vi "Keith 7001 Scan Example.vi"() -> ()   [LabVIEW 2019]
doc: "This is an example VI for the Keithley 7001 Switch System. The VI allows the operator to specify which cards are present and what channels are to be scanned. All the sources are set to immediate. The delay period applies to the trigger layer and occurs after each channel in the list is closed. After all the channels in the list have been closed, the 7001 will return to idle.\n By default this example scans channels 1 to 10 on card 1 with a 1 second delay after each channel closure."
uses:
  Keith 7001 Open/Close Chan.vi
panel:
  in  "delay period (sec)":dbl=1.0 min=0.0 max=99999.999 format="%.3f"
  out "error out":T1
  in  "error in":T1
  in  "channel list":T2(array[cluster])=[{"slot/memory"=1, "channel/row"=1, "column"=1, FALSE, FALSE}, {"slot/memory"=1, "channel/row"=2, "column"=1, FALSE, FALSE}, {"slot/memory"=1, "channel/row"=3, "column"=1, FALSE, FALSE}, {"slot/memory"=1, "channel/row"=4, "column"=1, FALSE, FALSE}, {"slot/memory"=1, "channel/row"=5, "column"=1, FALSE, FALSE}, {"slot/memory"=1, "channel/row"=6, "column"=1, FALSE, FALSE}, {"slot/memory"=1, "channel/row"=7, "column"=1, FALSE, FALSE}, {"slot/memory"=1, "channel/row"=8, "column"=1, FALSE, FALSE}, {"slot/memory"=1, "channel/row"=9, "column"=1, FALSE, FALSE}, {"slot/memory"=1, "channel/row"=10, "column"=1, FALSE, FALSE}] {"column" min=1; "channel/row" min=1; "slot/memory" min=1 max=2}
  in  "slot 2 card type (default:0)":u16(ring) items=["default", "none", "7052", "7053", "7054", "7056", "7057", "7058", "7062", "7063", "7064", "7065", "7066", "7067", "7154", "7156", "7158", "7164", "7166", "7168", "9990", "9991"]
  in  "slot 1 card type (default:0)":u16(ring) items=["default", "none", "7052", "7053", "7054", "7056", "7057", "7058", "7062", "7063", "7064", "7065", "7066", "7067", "7154", "7156", "7158", "7164", "7166", "7168", "9990", "9991"]
  in  "GPIB address":string="7"
  # "© Copyright 1993 National Instruments Corporation.  All Rights Reserved."
  # "memory location\nstandard channel"
  # "matrix card\nnon-matrix card"
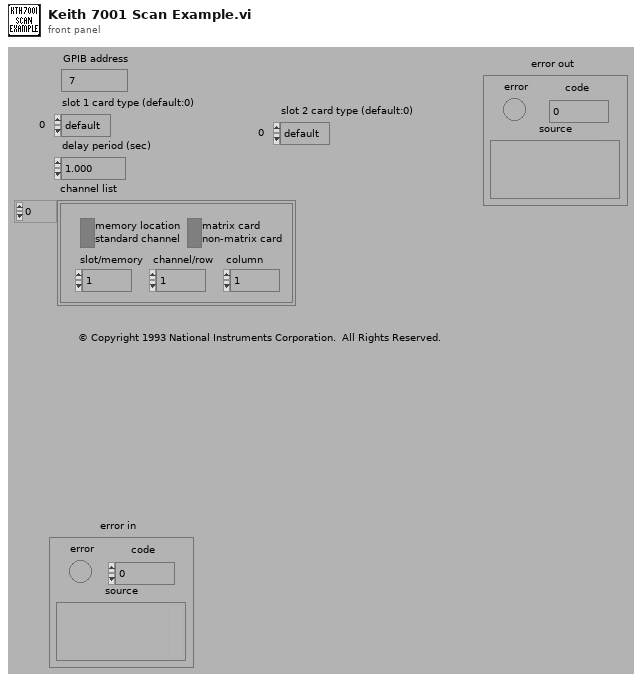
[diagram p1: front panel]
types:
  T1 = cluster{"error":bool, "code":i32, "source":string}
  T2 = cluster{"slot/memory":i16, "channel/row":i16, "column":i16, bool, bool}[]
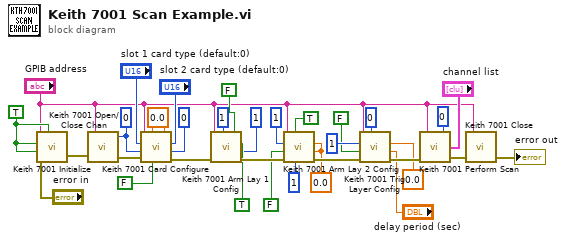
[diagram p0: block diagram]
diagram:
  w13 = 0.0
  w30 = 0.0
  w20 = u16 0
  w10 = TRUE
  n1 = call "Keith 7001 Initialize.vi"("GPIB address in"="GPIB address", "ID query"=w10, "reset"=w10, "error in"="error in", "error query"=w10) -> ("error out"=w22:T1)  [unwired: 1 out]
  n2 = call "Keith 7001 Open/Close Chan.vi"("GPIB address"="GPIB address", "error in"=w22, "open/close (open all:0)"=w20) -> ("error out"=w21:T1)  [unwired: 1 in]
  n3 = call "Keith 7001 Card Configure.vi"("slot 2 # of poles (default:0)"=u16 0, "slot 2 card type (default:0)"="slot 2 card type (default:0)", "slot 2 delay (sec)"=w30, "card pairing"=FALSE, "slot 1 delay (sec)"=w30, "error in"=w21, "slot 1 # of poles (default:0)"=w20, "slot 1 card type (default:0)"="slot 1 card type (default:0)", "GPIB address"="GPIB address") -> ("error out"=w31:T1)
  n4 = call "Keith 7001 Arm Lay 1 Config.vi"("count value"=u16 1, "count"=TRUE, "source bypass"=FALSE, "source (immediate:1)"=u16 1, "error in"=w31, "GPIB address"="GPIB address") -> ("error out"=w33:T1)  [unwired: 2 in]
  n5 = call "Keith 7001 Arm Lay 2 Config.vi"("delay period (sec)"=w13, "timer interval (sec)"=w13, "count value"=u16 1, "count"=TRUE, "error in"=w33, "source bypass"=FALSE, "source (immediate:1)"=u16 1, "GPIB address"="GPIB address") -> ("error out"=w32:T1)  [unwired: 2 in]
  n6 = call "Keith 7001 Trig Layer Config.vi"("delay period (sec)"="delay period (sec)", "timer interval (sec)"=0.0, "count (auto:0)"=u16 0, "error in"=w32, "source bypass"=FALSE, "source (immediate:1)"=u16 1, "GPIB address"="GPIB address") -> ("error out"=w24:T1)  [unwired: 3 in]
  n7 = call "Keith 7001 Perform Scan.vi"("GPIB address"="GPIB address", "error in"=w24, "scan options (arm, scan once:0)"=u16 0, "scan list"="channel list") -> ("error out"=w6:T1)
  n8 = call "Keith 7001 Close.vi"("error in"=w6, "GPIB address"="GPIB address") -> ("error out"=→"error out":T1)  [unwired: 1 in]
